vi "GetFFTDataSetProps.vi"(6 "do not write to database":bool, 8 "error in (no error)":errorcluster, 10 "MCSA FFT":T1, 11 "dataset props in":T2[](array[typedef])) -> (0 "error out":errorcluster, 3 "dataset props out":T2[](array[typedef]))   [LabVIEW 2017, in "McsaDataEventCreator.lvlib"]
uses:
  <vilib>/addons/InsightCM/Devices/Shared/Mcsa/McsaDataEventCreator/McsaDataEventCreator.lvlib
  <vilib>/addons/InsightCM/MessageBus/Base/controls/KeyValuePair.ctl
  <vilib>/addons/InsightCM/Utilities/Analysis/MCSA/controls/McsaFFT.ctl
  <vilib>/addons/InsightCM/Utilities/PropertyHelpers/PropertyHelpers.lvlib
  <vilib>/addons/InsightCM/Utilities/Analysis/MCSA/McsaAnalysisFunctions.lvlib
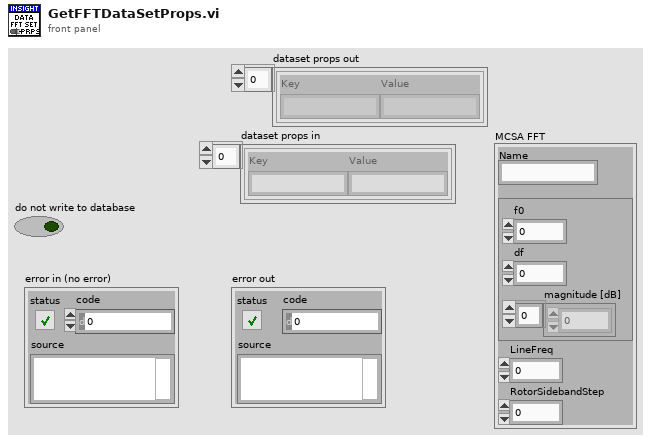
[diagram p1: front panel]
types:
  T1 = typedef "McsaAnalysisFunctions.lvlib/McsaFFT.ctl" = cluster{"Name":string, "Spectrum":cluster{"f0":dbl, "df":dbl, "magnitude [dB]":dbl[]}, "LineFreq":dbl, "RotorSidebandStep":dbl}
  T2 = typedef "KeyValuePair.ctl" = cluster{"Key":string, "Value":string}
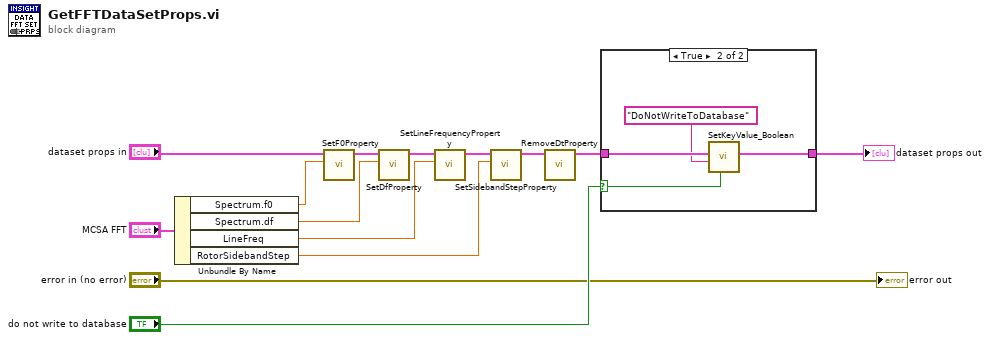
[diagram p0: block diagram]
diagram:
  n1 = Unbundle By Name("MCSA FFT") -> ("Spectrum.f0"=w6:dbl, "Spectrum.df"=w3:dbl, "LineFreq"=w5:dbl, "RotorSidebandStep"=w4:dbl)
  n2 = call <vilib>:"SetF0Property.vi"("F0"=w6, "props in"="dataset props in") -> ("props out"=w8:T2[])  [unwired: 9 in]
  n3 = call <vilib>:"SetDfProperty.vi"("df"=w3, "props in"=w8) -> ("props out"=w9:T2[])  [unwired: 9 in]
  n4 = call <vilib>:"SetLineFrequencyProperty.vi"("LineFrequency"=w5, "props in"=w9) -> ("props out"=w10:T2[])  [unwired: 9 in]
  n5 = call <vilib>:"SetSidebandStepProperty.vi"("RotorSidebandStep"=w4, "props in"=w10) -> ("props out"=w2:T2[])  [unwired: 9 in]
  n6 = call <vilib>:"RemoveDtProperty.vi"("props in"=w2) -> ("props out"=w1:T2[])  [unwired: 10 in]
  n7 = case shown="True" "do not write to database" {
    selector: "do not write to database" -> [_ w16]
    tunnel: w1 -> [w15 w19]
    tunnel: [w15 w18] -> w14
    frame False {
    }
    frame True {
      n8 = call <vilib>:"SetKeyValue_Boolean.vi"("value"=w16, "key"="DoNotWriteToDatabase", "key value pairs"=w19) -> ("key value pairs out"=w18:T2[])  [unwired: 8 in]
    }
  }
  "dataset props out" <- w14
  "error out" <- "error in (no error)"
